vi "Get All Channel Gains.vi"(8 "error in (no error)":errorcluster, 11 "Channel Params []":T1[](array[typedef])) -> (0 "error out":errorcluster, 3 "Gains []":dbl[](array[numeric]))   [LabVIEW 2019, in "KH7008.lvlib"]
uses:
  KH7008.lvlib
  typedefs/SetAll--Cluster.ctl
  typedefs/Channel--Enum.ctl
  typedefs/Gain--Enum.ctl
  typedefs/Input Configuration--Enum.ctl
  typedefs/Shunt--Enum.ctl
  typedefs/Coupling--Enum.ctl
  typedefs/Filter--Enum.ctl
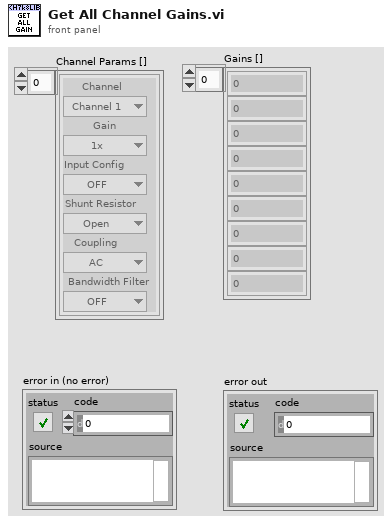
[diagram p1: front panel]
types:
  T1 = typedef "KH7008.lvlib/SetAll--Cluster.ctl" = cluster{"Channel":T2, "Gain":T3, "Input Config":T4, "Shunt Resistor":T5, "Coupling":T6, "Bandwidth Filter":T7}
  T2 = typedef "KH7008.lvlib/Channel--Enum.ctl" = enum8{"Channel 1", "Channel 2", "Channel 3", "Channel 4", "Channel 5", "Channel 6", "Channel 7", "Channel 8"}
  T3 = typedef "KH7008.lvlib/Gain--Enum.ctl" = enum8{"1x", "10x", "100x", "1000x"}
  T4 = typedef "KH7008.lvlib/Input Configuration--Enum.ctl" = enum8{"OFF", "SE+", "SE-", "DIFF"}
  T5 = typedef "KH7008.lvlib/Shunt--Enum.ctl" = enum8{"Open", "50 Ohms", "500 Ohms", "5k Ohms", "50k Ohms", "10M Ohm"}
  T6 = typedef "KH7008.lvlib/Coupling--Enum.ctl" = enum8{"AC", "DC"}
  T7 = typedef "KH7008.lvlib/Filter--Enum.ctl" = enum8{"OFF", "ON"}
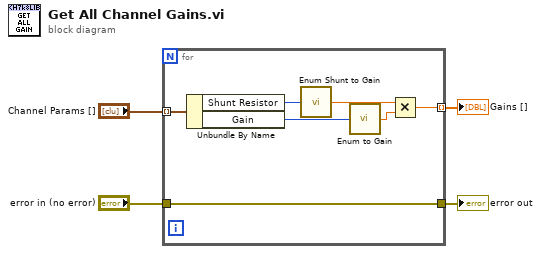
[diagram p0: block diagram]
diagram:
  n1 = for {
    tunnel: "Channel Params []" -> [w8] mode=indexing
    tunnel: [w11] -> w1 mode=indexing
    tunnel: "error in (no error)" -> [w5]
    tunnel: [w5] -> w3
    n2 = Unbundle By Name(w8) -> ("Shunt Resistor"=w7:T5, "Gain"=w6:T3)
    n3 = call "Enum Shunt to Gain.vi"("Shunt Resistor"=w7) -> ("Gain (V/A)"=w10:dbl)
    n4 = call "Enum to Gain.vi"("Gain"=w6) -> ("Gain (x)"=w9:dbl)
    n5 = Multiply(x=w10, y=w9) -> (x*y=w11:dbl)
  }
  "error out" <- w3
  "Gains []" <- w1
